vi "save_avg_image.vi"(8 "error in (no error)":errorcluster, 10 "Image":T1, 11 "ExperimentVariables in":refnum<class "ExperimentVariables.lvclass">) -> (0 "error out":errorcluster, 2 "Image Out (duplicate)":T1, 3 "ExperimentVariables out":refnum<class "ExperimentVariables.lvclass">)   [LabVIEW 2012]
uses:
  ExperimentVariables/ExperimentVariables.lvclass
  <vilib>/vision/Image Controls.llb/IMAQ Image.ctl
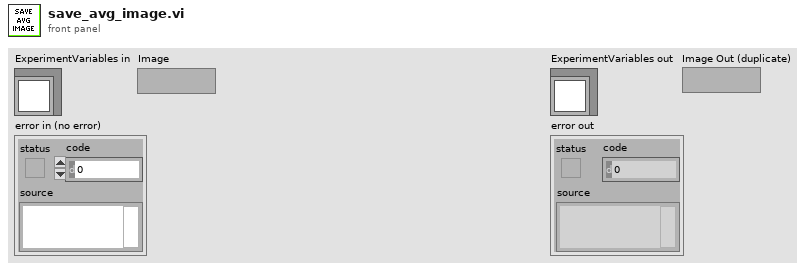
[diagram p1: front panel]
types:
  T1 = typedef "IMAQ Image.ctl" = refnum<image>
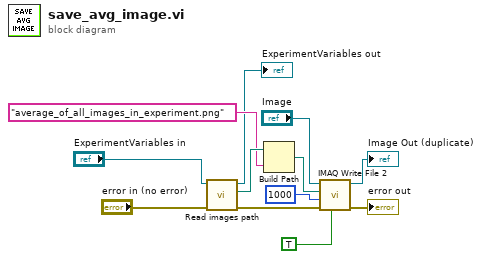
[diagram p0: block diagram]
diagram:
  n1 = call-dynamic "Read images path.vi"("error in (no error)"="error in (no error)", "ExperimentVariables in"="ExperimentVariables in") -> ("error out"=w4:errorcluster, "images path"=w12:path, "ExperimentVariables out"=→"ExperimentVariables out":refnum<class "ExperimentVariables.lvclass">)  [unwired: 7 in]
  n2 = Build Path(base path=w12, name or relative path="average_of_all_images_in_experiment.png") -> (appended path=w10:path)
  n3 = call-poly "IMAQ Write File 2"("Use bit depth? (false)"=TRUE, "error in (no error)"=w4, "Image Quality"=u32 1000, "File Path"=w10, "Image"="Image") -> ("error out"=→"error out":errorcluster, "Image Out (duplicate)"=→"Image Out (duplicate)":T1)  [unwired: 5 in]
